vi "Compute_Result.vi"(8 "error in (no error)":errorcluster, 10 "Autotest?":bool, 11 "Actor_Autotest in":refnum<class "Actor_Autotest.lvclass">) -> (0 "error out":errorcluster, 3 "Actor_Autotest out":refnum<class "Actor_Autotest.lvclass">)   [LabVIEW 2020, in "Library Core.lvlib" / "Actor_Autotest.lvlib" / "Actor_Autotest.lvclass"]
uses:
  Actor_Autotest.lvclass
  C:/Program Files (x86)/National Instruments/LabVIEW 2020/vi.lib/ActorFramework/Actor/Actor.lvclass
  Actor_Autotest.lvclass/Actor_Autotest.ctl
  Actor_Log/Actor_Log/Actor_Log Messages/Log Msg/Log Msg.lvclass/Log Msg.ctl
  <vilib>/ActorFramework/Message Enqueuer/Message Enqueuer.lvclass/Message Enqueuer.ctl
  <vilib>/ActorFramework/Actor/Actor.lvclass/Actor.ctl
  Instrument/Instrument (Default)/Class Instrument (Default).lvclass
  Commun VI/TypeDef/Commande Popup autotest/Commande element autotest.ctl
  <vilib>/ActorFramework/Message Enqueuer/Enqueue.vi
  <vilib>/ActorFramework/Message Enqueuer/Init from Existing Queue.vi
  Actor_Log/Actor_Log/Actor_Log Messages/Log Msg/Log Msg.lvclass
  C:/Program Files (x86)/National Instruments/LabVIEW 2020/vi.lib/ActorFramework/Message/Message.lvclass
  <vilib>/ActorFramework/Stop Msg/Stop Msg.lvclass
  <vilib>/ActorFramework/Message Priority Queue/Priority Enqueue.vi
  <vilib>/ActorFramework/Message Enqueuer/Message Enqueuer.lvclass
  Actor_Autotest Messages/Autotest_Result Msg/Autotest_Result Msg.lvclass
  <vilib>/ActorFramework/Actor/Actor.lvclass
panel:
  # "This VI send back the autotest result and close the actor by sending a close message"
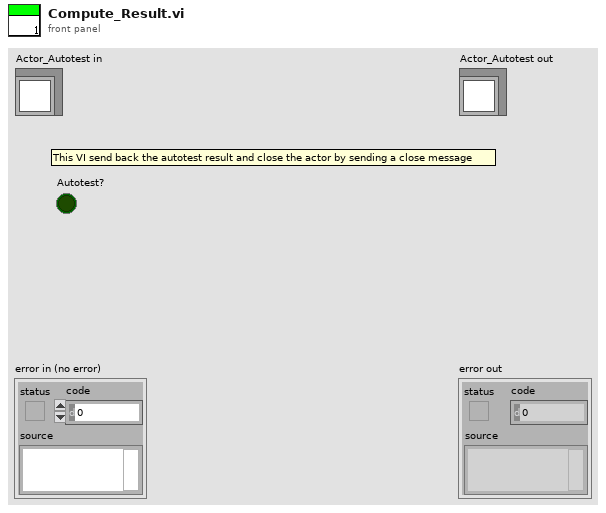
[diagram p1: front panel]
types:
  T1 = typedef "Commande element autotest.ctl" = cluster{"Instrument":string, "Etat":cluster{"Menu déroulant":u16}}
  T2 = cluster{"Instrument":refnum<class "Class Instrument (Default).lvclass">, "Element autotest":T1}
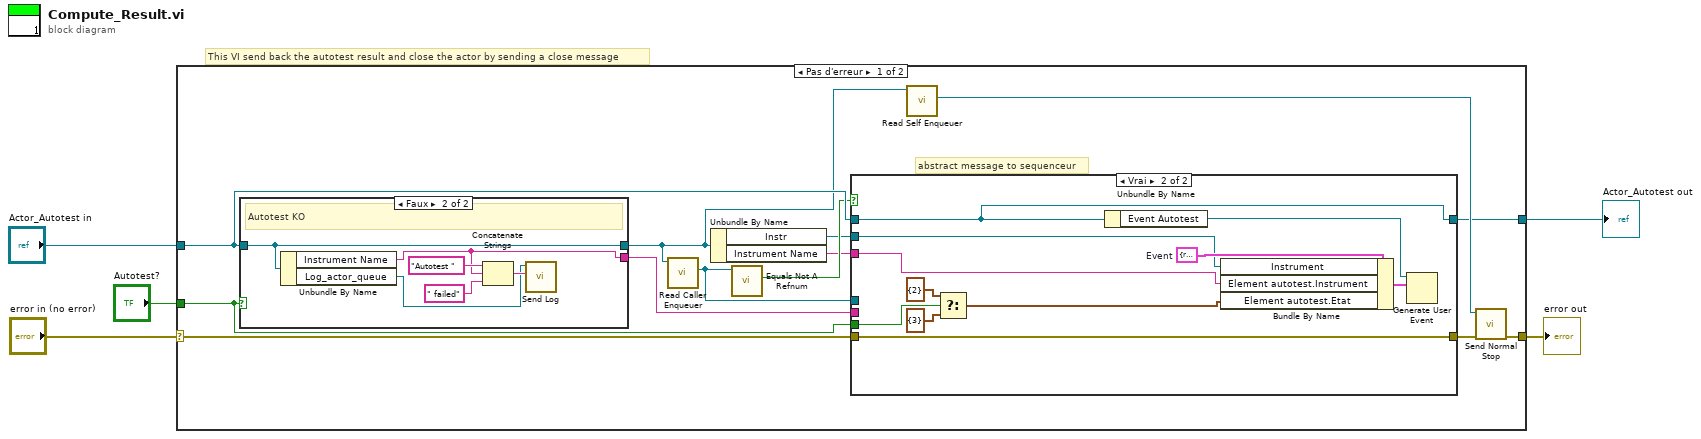
[diagram p0: block diagram]
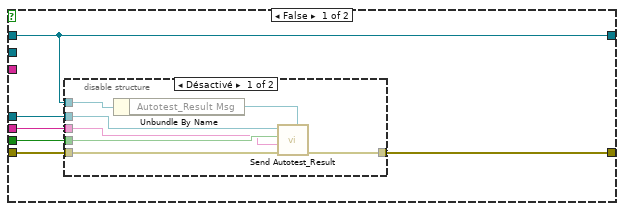
[diagram p2: hidden frame]
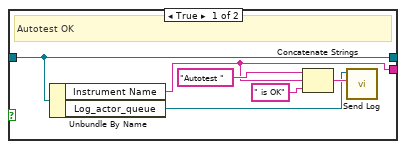
[diagram p4: hidden frame]
diagram:
  # "This VI send back the autotest result and close the actor by sending a close message"
  n1 = case shown="Pas d'erreur" "error in (no error)" {
    selector: "error in (no error)" -> [w17 w55]
    tunnel: [w18 w55] -> w4
    tunnel: [w9 w56] -> w2
    tunnel: "Actor_Autotest in" -> [w13 w56]
    tunnel: "Autotest?" -> [w15 _]
    frame No Error {
      # "abstract message to sequenceur"
      n2 = case shown="Faux" w15 {
        tunnel: w13 -> [w44 w50]
        tunnel: [w44 w50] -> w8
        tunnel: [w43 w49] -> w14
        frame True {
          # "Autotest OK"
          n3 = Unbundle By Name(w44) -> ("Instrument Name"=w43:string, "Log_actor_queue"=w45:refnum<class "Message Enqueuer.lvclass">)
          n4 = Concatenate Strings("Autotest ", w43, " is OK" ("string")) -> (w46:string)
          n5 = call "Send Log.vi"("String to add"=w46, "Message Enqueuer"=w45) -> ()  [unwired: 8 in, 2 out]
        }
        frame False {
          # "Autotest KO"
          n6 = Unbundle By Name(w50) -> ("Instrument Name"=w49:string, "Log_actor_queue"=w51:refnum<class "Message Enqueuer.lvclass">)
          n7 = Concatenate Strings("Autotest ", w49, " failed" ("string")) -> (w52:string)
          n8 = call "Send Log.vi"("String to add"=w52, "Message Enqueuer"=w51) -> ()  [unwired: 8 in, 2 out]
        }
      }
      n9 = call <vilib>:"Read Caller Enqueuer.vi"("Actor"=w8) -> ("Caller Enqueuer"=w11:refnum<class "Message Enqueuer.lvclass">)  [unwired: 10 in]
      n10 = Unbundle By Name(w8) -> ("Instr"=w7:refnum<class "Class Instrument (Default).lvclass">, "Instrument Name"=w6:string)
      n11 = call <vilib>:"Equals Not A Refnum.vi"("Message Enqueuer"=w11) -> ("Not a refnum?"=w10:bool)  [unwired: 10 in]
      n12 = case shown="Vrai" w10 {
        tunnel: w17 -> [w24 w42]
        tunnel: [w23 w42] -> w16
        tunnel: w15 -> [w22 w33]
        tunnel: w14 -> [w21 _]
        tunnel: w13 -> [w19 w41]
        tunnel: w11 -> [w20 _]
        tunnel: [w19 w41] -> w9
        tunnel: w7 -> [_ w38]
        tunnel: w6 -> [_ w37]
        frame False {
          n13 = disable-structure shown="Désactivé" {
            disable-tunnel: w24 -> [w31 _]
            disable-tunnel: [w30 _] -> w23
            disable-tunnel: w22 -> [w29 _]
            disable-tunnel: w21 -> [w28 _]
            disable-tunnel: w20 -> [w26 _]
            disable-tunnel: w19 -> [w25 _]
            frame Disabled {
              n14 = Unbundle By Name(w25) -> ("Autotest_Result Msg"=w27:refnum<class "Autotest_Result Msg.lvclass">)
              n15 = call "Send Autotest_Result.vi"("Message Type"=w27, "error in (no error)"=w31, "Instr"=w28, "Autotest"=w29, "Message Enqueuer"=w26) -> ("error out"=w30:errorcluster)  [unwired: 5 in, 1 out]
            }
            frame Enabled {
            }
          }
        }
        frame True {
          w39 = T2 {"Instrument"=refnum, "Element autotest"={"Instrument"="", "Etat"={"Menu déroulant"=0}}}  # Event
          n16 = Select(t=cluster{"Menu déroulant":u16} {"Menu déroulant"=2} ("Element autotest.Etat"), s=w33, f=cluster{"Menu déroulant":u16} {"Menu déroulant"=3} ("Element autotest.Etat")) -> (s? t:f=w32:cluster{"Menu déroulant":u16})
          n17 = Unbundle By Name(w41) -> ("Event Autotest"=w40:refnum<user-event>)
          n18 = Bundle By Name(cluster=w39, "Instrument"=w38, "Element autotest.Instrument"=w37, "Element autotest.Etat"=w32) -> (w36:T2)
          n19 = Generate User Event(user event=w40, event data cluster=w36) -> ()  [unwired: 2 in, 2 out]
        }
      }
      n20 = call <vilib>:"Read Self Enqueuer.vi"("Actor"=w8) -> ("Self Enqueuer"=w12:refnum<class "Message Enqueuer.lvclass">)  [unwired: 10 in]
      n21 = call <vilib>:"Send Normal Stop.vi"("error in (no error)"=w16, "Message Enqueuer"=w12) -> ("error out"=w18:errorcluster)  [unwired: 9 in]
    }
    frame Error {
    }
  }
  "error out" <- w4
  "Actor_Autotest out" <- w2
